vi "Perform Action Core.vi"(8 "error in (no error)":errorcluster, 11 "NI DAQmx AI Voltage in":refnum<class "NI DAQmx AI Voltage.lvclass">) -> (0 "error out":errorcluster, 3 "NI DAQmx AI Voltage out":refnum<class "NI DAQmx AI Voltage.lvclass">)   [LabVIEW 2023, in "NI DAQmx AI Voltage.lvlib" / "NI DAQmx AI Voltage.lvclass"]
uses:
  NI DAQmx AI Voltage.lvclass
  NI DAQmx AI Voltage.lvclass/NI DAQmx AI Voltage.ctl
  Device/Device/Device.lvclass
  D:/2_GitHub/LabVIEW-Device/Device/Device/Device.lvclass
  C:/Program Files (x86)/National Instruments/LabVIEW 2023/vi.lib/ActorFramework/Actor/Actor.lvclass
  D:/2_GitHub/LabVIEW-Device/Device Driver/NI DAQmx AI Voltage/NI DAQmx AI Voltage/NI DAQmx AI Voltage.lvclass
  <vilib>/DAQmx/read.llb/DAQmx Read (Analog 1D Wfm NChan NSamp).vi
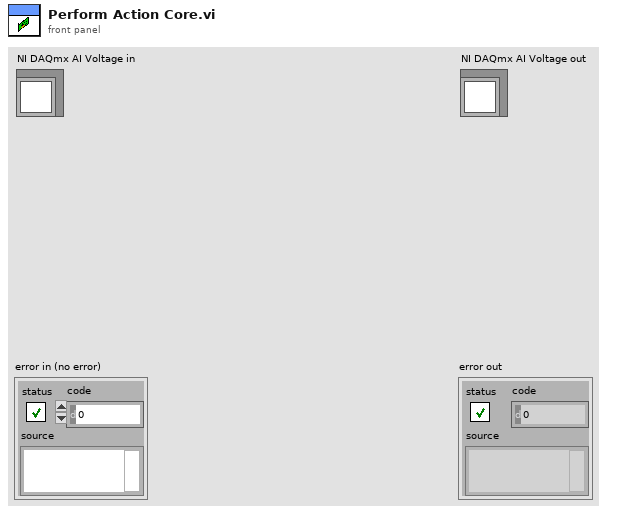
[diagram p1: front panel]
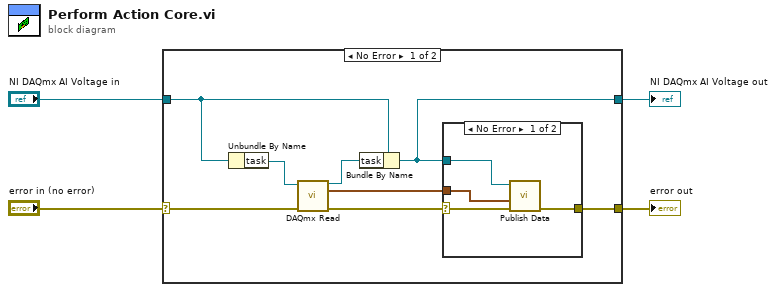
[diagram p0: block diagram]
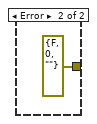
[diagram p2: hidden frame]
diagram:
  n1 = case shown="No Error" "error in (no error)" {
    selector: "error in (no error)" -> [w12 w19]
    tunnel: "NI DAQmx AI Voltage in" -> [w8 w18]
    tunnel: [w5 w19] -> w2
    tunnel: [w6 w18] -> w1
    frame No Error {
      n2 = Unbundle By Name(w8) -> ("task"=w11:refnum<k21>)
      n3 = call-poly <vilib>:"DAQmx Read.vi"("task/channels in"=w11, "error in"=w12) -> ("task out"=w7:refnum<k21>, "data"=w9:waveform(dbl)[], "error out"=w10:errorcluster)  [unwired: 11 in]
      n4 = Bundle By Name(cluster=w8, "task"=w7) -> (w6:refnum<class "NI DAQmx AI Voltage.lvclass">)
      n5 = case shown="No Error" w10 {
        selector: w10 -> [w16 _]
        tunnel: w9 -> [w14 _]
        tunnel: w6 -> [w15 _]
        tunnel: [w13 errorcluster {"status"=FALSE, "code"=0, "source"=""} ("error out")] -> w5
        frame No Error {
          n6 = call "Publish Data.vi"("error in (no error)"=w16, "waveform"=w14, "Device in"=w15) -> ("error out"=w13:errorcluster)  [unwired: 7 in, 1 out]
        }
        frame Error {
        }
      }
    }
    frame Error {
    }
  }
  "error out" <- w2
  "NI DAQmx AI Voltage out" <- w1
